vi "Timer.vi"(8 "error constant":errorcluster, 10 "Enum":enum16{"Reset", "Run", "Pause"}(ring)=enum."Run", 11 "Treshold":dbl format="%#_13g") -> (0 "error constant 2":errorcluster, 2 "Treshold":bool, 3 "Stoper":dbl)   [LabVIEW 2015]
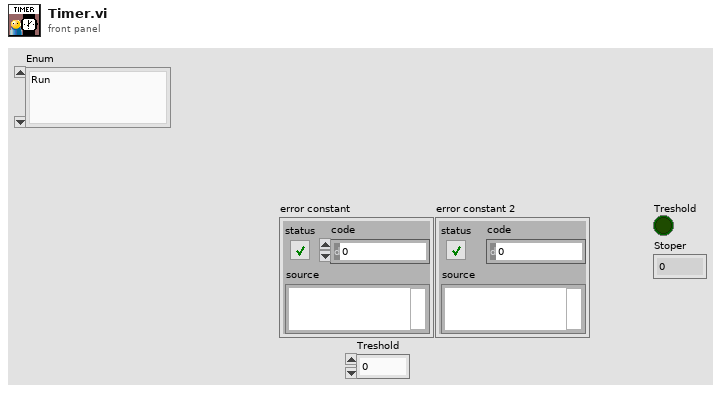
[diagram p1: front panel]
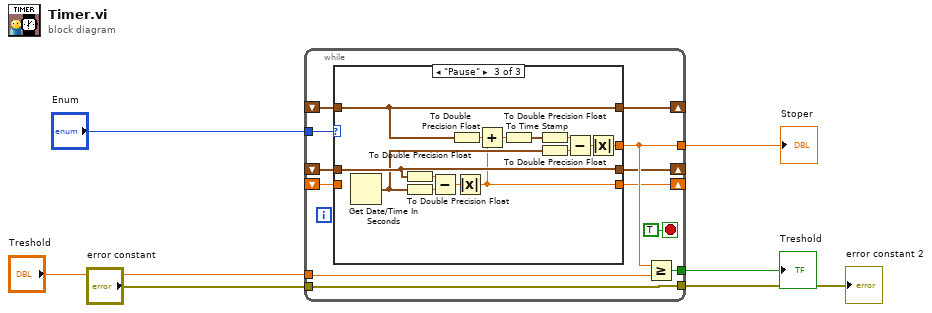
[diagram p0: block diagram]
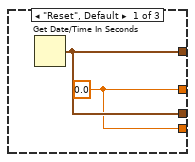
[diagram p2: hidden frame]
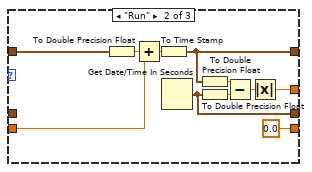
[diagram p3: hidden frame]
diagram:
  n1 = while {
    tunnel: "Enum" -> [w17]
    tunnel: "error constant" -> [w16]
    tunnel: [w16] -> w4
    shift-right: [w15] -> _
    shift-left: _ -> [w14]
    tunnel: "Treshold" -> [w13]
    tunnel: [w12] -> w1
    tunnel: [w11] -> w2
    shift-right: [w10] -> _
    shift-left: _ -> [w9]
    shift-right: [w8] -> _
    shift-left: _ -> [w7]
    stop <- TRUE stop-if-true
    n2 = case shown="\"Pause\"" w17 {
      tunnel: [w20 w22 w32] -> w15
      tunnel: w14 -> [_ w23 w32]
      tunnel: [w19 w28 w36] -> w12
      tunnel: [w20 w27 w42] -> w10
      tunnel: w9 -> [_ _ w42]
      tunnel: [w19 0.0 w35] -> w8
      tunnel: w7 -> [_ w21 _]
      frame "Reset", Default {
        w19 = 0.0
        n3 = Get Date/Time In Seconds() -> (seconds since 1Jan1904=w20:timestamp)
      }
      frame "Run" {
        n4 = To Double Precision Float(number=w23) -> (double precision float=w25:dbl)
        n5 = Add(x=w25, y=w21) -> (x+y=w24:dbl)
        n6 = To Time Stamp(1:w24) -> (0:w22:timestamp)
        n7 = Get Date/Time In Seconds() -> (seconds since 1Jan1904=w27:timestamp)
        n8 = To Double Precision Float(number=w22) -> (double precision float=w30:dbl)
        n9 = To Double Precision Float(number=w27) -> (double precision float=w31:dbl)
        n10 = Subtract(x=w30, y=w31) -> (x-y=w29:dbl)
        n11 = Absolute Value(x=w29) -> (abs(x)=w28:dbl)
      }
      frame "Pause" {
        n12 = Get Date/Time In Seconds() -> (seconds since 1Jan1904=w38:timestamp)
        n13 = To Double Precision Float(number=w42) -> (double precision float=w44:dbl)
        n14 = To Double Precision Float(number=w38) -> (double precision float=w45:dbl)
        n15 = Subtract(x=w44, y=w45) -> (x-y=w43:dbl)
        n16 = To Double Precision Float(number=w32) -> (double precision float=w37:dbl)
        n17 = Absolute Value(x=w43) -> (abs(x)=w35:dbl)
        n18 = Add(x=w37, y=w35) -> (x+y=w34:dbl)
        n19 = To Time Stamp(1:w34) -> (0:w33:timestamp)
        n20 = To Double Precision Float(number=w33) -> (double precision float=w40:dbl)
        n21 = To Double Precision Float(number=w38) -> (double precision float=w39:dbl)
        n22 = Subtract(x=w40, y=w39) -> (x-y=w41:dbl)
        n23 = Absolute Value(x=w41) -> (abs(x)=w36:dbl)
      }
    }
    n24 = Greater Or Equal?(x=w12, y=w13) -> (x >= y?=w11:bool)
  }
  "error constant 2" <- w4
  "Treshold" <- w2
  "Stoper" <- w1
